vi "StartUp Sequence Open Loop Rev 1.2 -Retarded Engine Ramp Up.vi"() -> ()   [LabVIEW 2017]
panel:
  out "Turbine State 3":string
  out "Turbine State 2":string
  in  "Shut Off":bool
  out "ECU COM Port Out":refnum<visa-resource-name>
  out "Throttle Position":string
  out "Turbine RPM":string
  out "Turbine Temp":string
  out "Pump Voltage":string
  out "Error Out":errorcluster
  in  "Error In":errorcluster
  in  "ECU COM Port":refnum<visa-resource-name>
  out "Turbine State":string
  in  "Strt Sqnc":bool
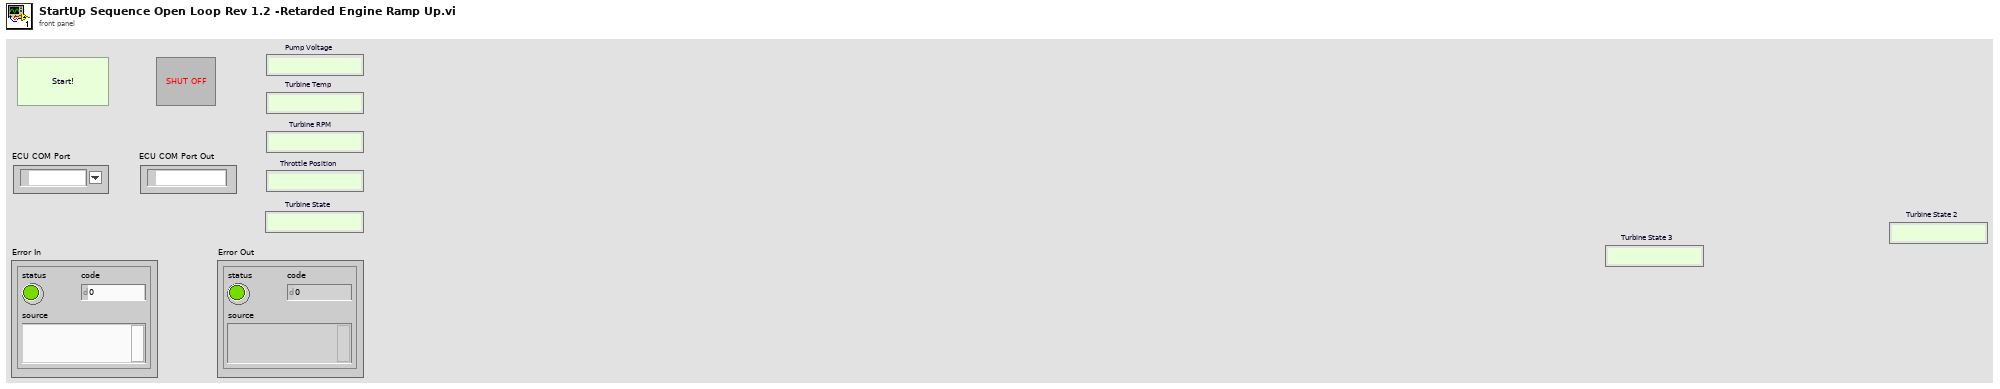
[diagram p1: front panel]
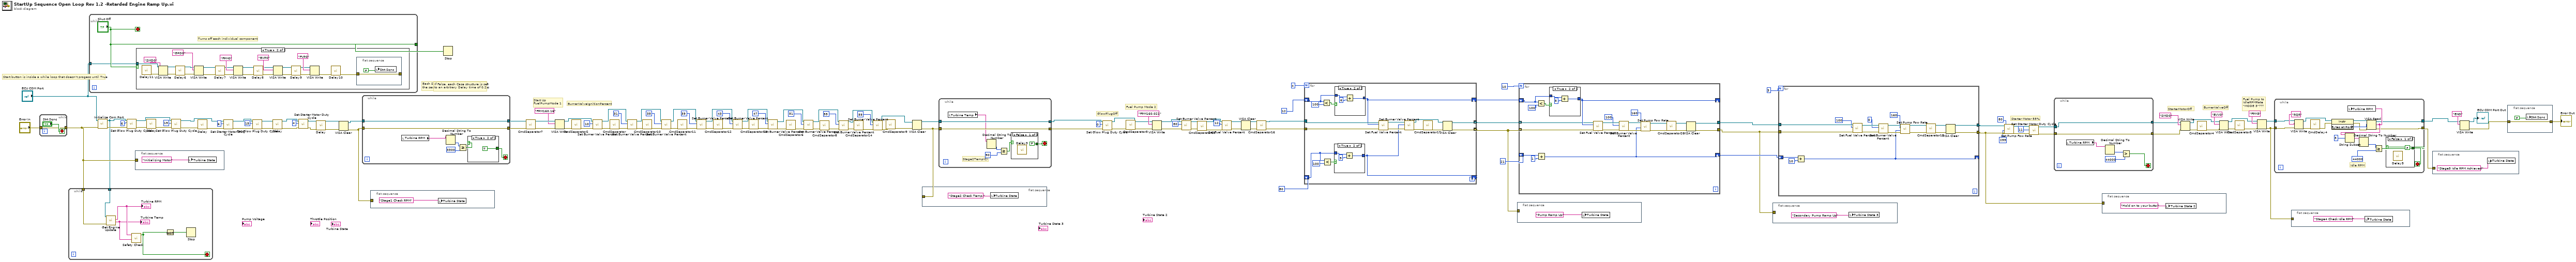
[diagram p0: block diagram]
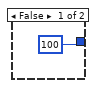
[diagram p2: hidden frame]
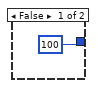
[diagram p3: hidden frame]
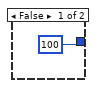
[diagram p4: hidden frame]
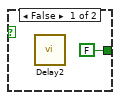
[diagram p6: hidden frame]
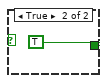
[diagram p7: hidden frame]
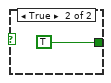
[diagram p8: hidden frame]
diagram:
  # "Starter Motor 55%"
  # "Start button is inside a while loop that doesn't progess until True"
  # "Fuel Pump Mode 2"
  # "Fuel Pump to \nIdleRPMRate\n\"MODE 3\"???"
  # "BurnerValveOff"
  # "StarterMotorOff"
  # "GlowPlugOff"
  # "Start Up\nFuelPumpMode 1"
  # "BurnerValveIgnitionPercent"
  # "If False, each Case structure is set\nto an arbitrary Delay time of 0.2 s"
  # "Each Stage is inside a while loop so that \nthe sequence doesn't progress until True"
  n1 = while {
    tunnel: "Error In" -> [w132]
    tunnel: [w132] -> w18
    stop <- "Strt Sqnc" stop-if-true
  }
  n2 = while {
    tunnel: ["Shut Off"] -> w104
    tunnel: "ECU COM Port" -> [w134]
    stop <- "Shut Off" stop-if-true
    # "Turns off each individual component"
    n3 = case shown="True" "Shut Off" {
      tunnel: w134 -> [_ w138]
      frame False {
      }
      frame True {
        n4 = call "Delay11"() -> ("error out"=w136:errorcluster)  [unwired: 11 in]
        n5 = VISA Write(VISA resource name=w138, write buffer="SMD0", error in (no error)=w136) -> (VISA resource name out=w143:refnum<visa-resource-name>, error out=w156:errorcluster)  [unwired: 1 out]
        n6 = call "Delay6"("error in (no error)"=w156) -> ("error out"=w150:errorcluster)  [unwired: 10 in]
        n7 = VISA Write(VISA resource name=w143, write buffer="GPD0", error in (no error)=w150) -> (VISA resource name out=w141:refnum<visa-resource-name>, error out=w154:errorcluster)  [unwired: 1 out]
        n8 = call "Delay7"("error in (no error)"=w154) -> ("error out"=w149:errorcluster)  [unwired: 10 in]
        n9 = VISA Write(VISA resource name=w141, write buffer="FPM0", error in (no error)=w149) -> (VISA resource name out=w140:refnum<visa-resource-name>, error out=w153:errorcluster)  [unwired: 1 out]
        n10 = call "Delay8"("error in (no error)"=w153) -> ("error out"=w148:errorcluster)  [unwired: 10 in]
        n11 = VISA Write(VISA resource name=w140, write buffer="BVP0", error in (no error)=w148) -> (VISA resource name out=w139:refnum<visa-resource-name>, error out=w152:errorcluster)  [unwired: 1 out]
        n12 = call "Delay9"("error in (no error)"=w152) -> ("error out"=w147:errorcluster)  [unwired: 10 in]
        n13 = VISA Write(VISA resource name=w139, write buffer="FVP0", error in (no error)=w147) -> (error out=w151:errorcluster)  [unwired: 2 out]
        n14 = call "Delay10"("error in (no error)"=w151) -> ("error out"=w137:errorcluster)  [unwired: 10 in]
        n15 = flat-sequence {
          tunnel: w137 -> [w157]
          tunnel: [w157] -> _
          frame #0 {
            n16 = local write "Strt Sqnc"(FALSE ("Strt Sqnc")) -> ()
          }
        }
      }
    }
  }
  n17 = call "Initialize Com Port.vi"("Error In"=w18, "ECU COM Port"="ECU COM Port") -> ("Error Out"=w92:errorcluster, "ECU COM Port Out"=w17:refnum<visa-resource-name>)  [unwired: 8 in]
  n18 = while {
    tunnel: w18 -> [w164]
    tunnel: w17 -> [w163]
    stop <- w160 stop-if-true
    n19 = call "Get Engine Update.vi"("Error In"=w164, "ECU COM Port"=w163) -> ("Temperature"=w161:string, "RPMs"=w162:string)  [unwired: 6 in, 2 out]
    "Turbine RPM" <- w162
    "Turbine Temp" <- w161
    n20 = call "Safety Check.vi"("Temperature"=w161, "RPMs"=w162) -> ("Safe?"=w160:bool)  [unwired: 9 in]
    n21 = Not(x=w160) -> (.not. x?=w159:bool)
    n22 = Stop(stop? (T)=w159) -> ()
  }
  n23 = call "Set Glow Plug Duty Cycle.vi"("Error In"=w92, "Duty Cycle"=6, "ECU COM Port"=w17) -> ("Error Out"=w91:errorcluster, "ECU COM Port Out"=w88:refnum<visa-resource-name>)  [unwired: 7 in]
  n24 = flat-sequence {
    tunnel: w18 -> [_]
    frame #0 {
      n25 = local write "Turbine State"("Initializing Motor") -> ()
    }
  }
  n26 = call "Delay"("error in (no error)"=w91) -> ("error out"=w90:errorcluster)  [unwired: 10 in]
  n27 = call "Set Glow Plug Duty Cycle.vi"("Error In"=w90, "Duty Cycle"=19, "ECU COM Port"=w88) -> ("Error Out"=w89:errorcluster, "ECU COM Port Out"=w84:refnum<visa-resource-name>)  [unwired: 7 in]
  n28 = call "Delay"("error in (no error)"=w89) -> ("error out"=w85:errorcluster)  [unwired: 10 in]
  n29 = call "Set Starter Motor Duty Cycle.vi"("Error In"=w85, "Duty Cycle"=6, "ECU COM Port"=w84) -> ("Error Out"=w83:errorcluster, "ECU COM Port Out"=w81:refnum<visa-resource-name>)  [unwired: 7 in]
  n30 = call "Set Glow Plug Duty Cycle.vi"("Error In"=w83, "Duty Cycle"=15, "ECU COM Port"=w81) -> ("Error Out"=w82:errorcluster, "ECU COM Port Out"=w77:refnum<visa-resource-name>)  [unwired: 7 in]
  n31 = call "Delay"("error in (no error)"=w82) -> ("error out"=w79:errorcluster)  [unwired: 10 in]
  n32 = call "Set Starter Motor Duty Cycle.vi"("Error In"=w79, "Duty Cycle"=4, "ECU COM Port"=w77) -> ("Error Out"=w78:errorcluster, "ECU COM Port Out"=w76:refnum<visa-resource-name>)  [unwired: 7 in]
  n33 = call "Delay"("error in (no error)"=w78) -> ("error out"=w107:errorcluster)  [unwired: 10 in]
  n34 = VISA Clear(VISA resource name=w76, error in (no error)=w107) -> (VISA resource name out=w108:refnum<visa-resource-name>, error out=w109:errorcluster)
  n35 = while {
    tunnel: w109 -> [w168]
    tunnel: w108 -> [w167]
    tunnel: [w167] -> w119
    tunnel: [w168] -> w118
    stop <- w171 stop-if-true
    n36 = local read "Turbine RPM"() -> (w166:string)
    n37 = Decimal String To Number(string=w166) -> (number=w170:i32)  [unwired: 2 in, 1 out]
    n38 = Greater Or Equal?(x=w170, y=3300) -> (x >= y?=w172:bool)
    n39 = case shown="True" w172 {
      tunnel: [FALSE TRUE] -> w171
      frame False {
        n40 = call "Delay2"() -> ()  [unwired: 11 in, 1 out]
      }
      frame True {
      }
    }
  }
  n41 = flat-sequence {
    tunnel: w109 -> [_]
    frame #0 {
      n42 = local write "Turbine State"("Stage1 Check RPM") -> ()
    }
  }
  n43 = Stop(stop? (T)=w104) -> ()
  n44 = call "CmdSeparator7"("error in (no error)"=w118) -> ("error out"=w117:errorcluster)  [unwired: 10 in]
  n45 = VISA Write(VISA resource name=w119, write buffer="FPM160,16", error in (no error)=w117) -> (VISA resource name out=w64:refnum<visa-resource-name>, error out=w130:errorcluster)  [unwired: 1 out]
  n46 = call "CmdSeparator2"("error in (no error)"=w130) -> ("error out"=w75:errorcluster)  [unwired: 10 in]
  n47 = call "Set Burner Valve Percent.vi"("Error In"=w75, "Percent"=10, "ECU COM Port"=w64) -> ("Error Out"=w74:errorcluster, "ECU COM Port Out"=w63:refnum<visa-resource-name>)  [unwired: 7 in]
  n48 = call "CmdSeparator"("error in (no error)"=w74) -> ("error out"=w73:errorcluster)  [unwired: 10 in]
  n49 = call "Set Burner Valve Percent.vi"("Error In"=w73, "Percent"=31, "ECU COM Port"=w63) -> ("Error Out"=w72:errorcluster, "ECU COM Port Out"=w62:refnum<visa-resource-name>)  [unwired: 7 in]
  n50 = call "CmdSeparator10"("error in (no error)"=w72) -> ("error out"=w71:errorcluster)  [unwired: 10 in]
  n51 = call "Set Burner Valve Percent.vi"("Error In"=w71, "Percent"=35, "ECU COM Port"=w62) -> ("Error Out"=w70:errorcluster, "ECU COM Port Out"=w61:refnum<visa-resource-name>)  [unwired: 7 in]
  n52 = call "CmdSeparator11"("error in (no error)"=w70) -> ("error out"=w69:errorcluster)  [unwired: 10 in]
  n53 = call "Set Burner Valve Percent.vi"("Error In"=w69, "Percent"=39, "ECU COM Port"=w61) -> ("Error Out"=w68:errorcluster, "ECU COM Port Out"=w60:refnum<visa-resource-name>)  [unwired: 7 in]
  n54 = call "CmdSeparator12"("error in (no error)"=w68) -> ("error out"=w67:errorcluster)  [unwired: 10 in]
  n55 = call "Set Burner Valve Percent.vi"("Error In"=w67, "Percent"=43, "ECU COM Port"=w60) -> ("Error Out"=w66:errorcluster, "ECU COM Port Out"=w59:refnum<visa-resource-name>)  [unwired: 7 in]
  n56 = call "CmdSeparator13"("error in (no error)"=w66) -> ("error out"=w65:errorcluster)  [unwired: 10 in]
  n57 = call "Set Burner Valve Percent.vi"("Error In"=w65, "Percent"=47, "ECU COM Port"=w59) -> ("Error Out"=w38:errorcluster, "ECU COM Port Out"=w37:refnum<visa-resource-name>)  [unwired: 7 in]
  n58 = call "CmdSeparator6"("error in (no error)"=w38) -> ("error out"=w40:errorcluster)  [unwired: 10 in]
  n59 = call "Set Burner Valve Percent.vi"("Error In"=w40, "Percent"=51, "ECU COM Port"=w37) -> ("Error Out"=w33:errorcluster, "ECU COM Port Out"=w34:refnum<visa-resource-name>)  [unwired: 7 in]
  n60 = call "CmdSeparator8"("error in (no error)"=w33) -> ("error out"=w36:errorcluster)  [unwired: 10 in]
  n61 = call "Set Burner Valve Percent.vi"("Error In"=w36, "Percent"=55, "ECU COM Port"=w34) -> ("Error Out"=w29:errorcluster, "ECU COM Port Out"=w30:refnum<visa-resource-name>)  [unwired: 7 in]
  n62 = call "CmdSeparator14"("error in (no error)"=w29) -> ("error out"=w32:errorcluster)  [unwired: 10 in]
  n63 = call "Set Burner Valve Percent.vi"("Error In"=w32, "Percent"=59, "ECU COM Port"=w30) -> ("Error Out"=w28:errorcluster, "ECU COM Port Out"=w27:refnum<visa-resource-name>)  [unwired: 7 in]
  n64 = call "CmdSeparator9"("error in (no error)"=w28) -> ("error out"=w103:errorcluster)  [unwired: 10 in]
  n65 = VISA Clear(VISA resource name=w27, error in (no error)=w103) -> (VISA resource name out=w105:refnum<visa-resource-name>, error out=w106:errorcluster)
  n66 = flat-sequence {
    tunnel: w106 -> [_]
    frame #0 {
      n67 = local write "Turbine State"("Stage2 Check Temp.") -> ()
    }
  }
  n68 = while {
    tunnel: w105 -> [w178]
    tunnel: w106 -> [w179]
    tunnel: [w178] -> w48
    tunnel: [w179] -> w49
    stop <- w182 stop-if-true
    # "Stage2Temp(C)"
    n69 = local read "Turbine Temp"() -> (w177:string)
    n70 = Decimal String To Number(string=w177) -> (number=w180:i32)  [unwired: 2 in, 1 out]
    n71 = Greater Or Equal?(x=w180, y=90) -> (x >= y?=w183:bool)
    n72 = case shown="False" w183 {
      tunnel: [FALSE TRUE] -> w182
      frame False {
        n73 = call "Delay3"() -> ()  [unwired: 11 in, 1 out]
      }
      frame True {
      }
    }
  }
  n74 = call "Set Glow Plug Duty Cycle.vi"("Error In"=w49, "Duty Cycle"=0, "ECU COM Port"=w48) -> ("Error Out"=w47:errorcluster, "ECU COM Port Out"=w45:refnum<visa-resource-name>)  [unwired: 7 in]
  n75 = call "CmdSeparator3"("error in (no error)"=w47) -> ("error out"=w46:errorcluster)  [unwired: 10 in]
  n76 = VISA Write(VISA resource name=w45, write buffer="FPM160,021", error in (no error)=w46) -> (VISA resource name out=w42:refnum<visa-resource-name>, error out=w44:errorcluster)  [unwired: 1 out]
  n77 = call "Set Burner Valve Percent.vi"("Error In"=w44, "Percent"=80, "ECU COM Port"=w42) -> ("Error Out"=w26:errorcluster, "ECU COM Port Out"=w41:refnum<visa-resource-name>)  [unwired: 7 in]
  n78 = call "CmdSeparator18"("error in (no error)"=w26) -> ("error out"=w25:errorcluster)  [unwired: 10 in]
  n79 = call "Set Fuel Valve Percent.vi"("Error In"=w25, "Percent"=12, "ECU COM Port"=w41) -> ("Error Out"=w24:errorcluster, "ECU COM Port Out"=w43:refnum<visa-resource-name>)  [unwired: 7 in]
  n80 = VISA Clear(VISA resource name=w43, error in (no error)=w24) -> (VISA resource name out=w99:refnum<visa-resource-name>, error out=w100:errorcluster)
  n81 = call "CmdSeparator16"("error in (no error)"=w100) -> ("error out"=w98:errorcluster)  [unwired: 10 in]
  n82 = for {
    N: 4 -> [_]
    tunnel: [w186] -> _
    tunnel: [w187] -> _
    tunnel: w99 -> [w194]
    tunnel: w98 -> [w195]
    shift-right: [w193] -> w20
    shift-left: 12 -> [w199]
    shift-right: [w190] -> _
    shift-left: 80 -> [w196]
    tunnel: [w187] -> w7 mode=indexing
    tunnel: [w186] -> w21 mode=indexing
    n83 = Less?(x=w199, y=100) -> (x < y?=w200:bool)
    n84 = Less?(x=w196, y=100) -> (x < y?=w197:bool)
    n85 = case shown="True" w197 {
      tunnel: w196 -> [_ w206]
      tunnel: [100 w204] -> w190
      frame False {
      }
      frame True {
        n86 = Add(x=w206, y=5) -> (x+y=w204:i32)
      }
    }
    n87 = case shown="True" w200 {
      tunnel: w199 -> [_ w210]
      tunnel: [100 w208] -> w193
      frame False {
      }
      frame True {
        n88 = Add(x=w210, y=6) -> (x+y=w208:i32)
      }
    }
    n89 = call "Set Fuel Valve Percent.vi"("Error In"=w195, "Percent"=w193, "ECU COM Port"=w194) -> ("Error Out"=w192:errorcluster, "ECU COM Port Out"=w189:refnum<visa-resource-name>)  [unwired: 7 in]
    n90 = call "Set Burner Valve Percent.vi"("Error In"=w192, "Percent"=w190, "ECU COM Port"=w189) -> ("Error Out"=w191:errorcluster, "ECU COM Port Out"=w188:refnum<visa-resource-name>)  [unwired: 7 in]
    n91 = call "CmdSeparator17"("error in (no error)"=w191) -> ("error out"=w202:errorcluster)  [unwired: 10 in]
    n92 = VISA Clear(VISA resource name=w188, error in (no error)=w202) -> (VISA resource name out=w186:refnum<visa-resource-name>, error out=w187:errorcluster)
  }
  n93 = flat-sequence {
    tunnel: w7 -> [_]
    frame #0 {
      n94 = local write "Turbine State"("Pump Ramp Up") -> ()
    }
  }
  n95 = for {
    N: 10 -> [_]
    tunnel: [w223] -> w15
    tunnel: [w224] -> w6
    shift-right: [w227] -> _
    shift-left: w20 -> [w228]
    tunnel: w7 -> [w222] mode=indexing
    tunnel: w21 -> [w221] mode=indexing
    shift-right: [w212] -> w14
    shift-left: 21 -> [w213]
    n96 = Less?(x=w228, y=100) -> (x < y?=w229:bool)
    n97 = Add(x=w213, y=1) -> (x+y=w212:i32)
    n98 = case shown="True" w229 {
      tunnel: w228 -> [_ w235]
      tunnel: [100 w233] -> w227
      frame False {
      }
      frame True {
        n99 = Add(x=w235, y=5) -> (x+y=w233:i32)
      }
    }
    n100 = call "Set Fuel Valve Percent.vi"("Error In"=w222, "Percent"=w227, "ECU COM Port"=w221) -> ("Error Out"=w226:errorcluster, "ECU COM Port Out"=w225:refnum<visa-resource-name>)  [unwired: 7 in]
    n101 = call "Set Burner Valve Percent.vi"("Error In"=w226, "Percent"=100 ("y"), "ECU COM Port"=w225) -> ("Error Out"=w216:errorcluster, "ECU COM Port Out"=w219:refnum<visa-resource-name>)  [unwired: 7 in]
    n102 = call "Set Pump Fow Rate.vi"("Error In"=w216, "Pulse Width"=w212, "Voltage"=160 ("y"), "ECU COM Port"=w219) -> ("Error Out"=w217:errorcluster, "ECU COM Port Out"=w218:refnum<visa-resource-name>)  [unwired: 6 in]
    n103 = call "CmdSeparator20"("error in (no error)"=w217) -> ("error out"=w231:errorcluster)  [unwired: 10 in]
    n104 = VISA Clear(VISA resource name=w218, error in (no error)=w231) -> (VISA resource name out=w223:refnum<visa-resource-name>, error out=w224:errorcluster)
  }
  n105 = flat-sequence {
    tunnel: w6 -> [_]
    frame #0 {
      n106 = local write "Turbine State 3"("Secondary Pump Ramp Up") -> ()
    }
  }
  n107 = for {
    N: 3 -> [_]
    tunnel: [w249] -> w10
    tunnel: [w250] -> w5
    tunnel: w6 -> [w248]
    tunnel: w15 -> [w247]
    shift-right: [w238] -> _
    shift-left: w14 -> [w239]
    n108 = Add(x=w239, y=10) -> (x+y=w238:i32)
    n109 = call "Set Fuel Valve Percent.vi"("Error In"=w248, "Percent"=100 ("y"), "ECU COM Port"=w247) -> ("Error Out"=w252:errorcluster, "ECU COM Port Out"=w251:refnum<visa-resource-name>)  [unwired: 7 in]
    n110 = call "Set Burner Valve Percent.vi"("Error In"=w252, "Percent"=0 ("y"), "ECU COM Port"=w251) -> ("Error Out"=w242:errorcluster, "ECU COM Port Out"=w245:refnum<visa-resource-name>)  [unwired: 7 in]
    n111 = call "Set Pump Fow Rate.vi"("Error In"=w242, "Pulse Width"=w238, "Voltage"=160 ("y"), "ECU COM Port"=w245) -> ("Error Out"=w243:errorcluster, "ECU COM Port Out"=w244:refnum<visa-resource-name>)  [unwired: 6 in]
    n112 = call "CmdSeparator15"("error in (no error)"=w243) -> ("error out"=w253:errorcluster)  [unwired: 10 in]
    n113 = VISA Clear(VISA resource name=w244, error in (no error)=w253) -> (VISA resource name out=w249:refnum<visa-resource-name>, error out=w250:errorcluster)
  }
  n114 = call "Set Pump Fow Rate.vi"("Error In"=w5, "Pulse Width"=255, "Voltage"=80, "ECU COM Port"=w10) -> ("Error Out"=w11:errorcluster, "ECU COM Port Out"=w12:refnum<visa-resource-name>)  [unwired: 6 in]
  n115 = call "Set Starter Motor Duty Cycle.vi"("Error In"=w11, "Duty Cycle"=11, "ECU COM Port"=w12) -> ("Error Out"=w4:errorcluster, "ECU COM Port Out"=w3:refnum<visa-resource-name>)  [unwired: 7 in]
  n116 = while {
    tunnel: w4 -> [w255]
    tunnel: w3 -> [w254]
    tunnel: [w255] -> w2
    tunnel: [w254] -> w1
    stop <- w256 stop-if-true
    n117 = local read "Turbine RPM"() -> (w259:string)
    n118 = Decimal String To Number(string=w259) -> (number=w258:i32)  [unwired: 2 in, 1 out]
    n119 = Greater?(x=w258, y=44000) -> (0:w256:bool)
  }
  n120 = flat-sequence {
    tunnel: w5 -> [_]
    frame #0 {
      n121 = local write "Turbine State 2"("Hold on to your butts!") -> ()
    }
  }
  n122 = VISA Write(VISA resource name=w1, write buffer="SMD0", error in (no error)=w2) -> (VISA resource name out=w125:refnum<visa-resource-name>, error out=w127:errorcluster)  [unwired: 1 out]
  n123 = call "CmdSeparator4"("error in (no error)"=w127) -> ("error out"=w126:errorcluster)  [unwired: 10 in]
  n124 = VISA Write(VISA resource name=w125, write buffer="BVV0", error in (no error)=w126) -> (VISA resource name out=w122:refnum<visa-resource-name>, error out=w121:errorcluster)  [unwired: 1 out]
  n125 = call "CmdSeparator5"("error in (no error)"=w121) -> ("error out"=w123:errorcluster)  [unwired: 10 in]
  n126 = VISA Write(VISA resource name=w122, write buffer="FPM3", error in (no error)=w123) -> (VISA resource name out=w120:refnum<visa-resource-name>, error out=w111:errorcluster)  [unwired: 1 out]
  n127 = while {
    tunnel: w120 -> [w267]
    tunnel: w111 -> [w266]
    tunnel: [w264] -> w110
    tunnel: [w263] -> w113
    stop <- w278 stop-if-true
    # "Idle RPM"
    n128 = VISA Write(VISA resource name=w267, write buffer="RQR", error in (no error)=w266) -> (VISA resource name out=w274:refnum<visa-resource-name>, error out=w276:errorcluster)  [unwired: 1 out]
    n129 = call "CmdDelay4"("error in (no error)"=w276) -> ("error out"=w275:errorcluster)  [unwired: 10 in]
    n130 = property class="Instr"(reference=w274, error in=w275) -> (reference out=w271:refnum<visa-resource-name>, error out=w272:errorcluster, "Bytes at Port"=w273:u32)
    n131 = VISA Read(VISA resource name=w271, byte count=w273, error in (no error)=w272) -> (VISA resource name out=w263:refnum<visa-resource-name>, read buffer=w265:string, error out=w264:errorcluster)  [unwired: 1 out]
    n132 = String Subset(string=w265, offset (0)=3) -> (substring=w269:string)  [unwired: 1 in]
    n133 = local write "Turbine RPM"(w265) -> ()
    n134 = Decimal String To Number(string=w269) -> (number=w268:i32)  [unwired: 2 in, 1 out]
    n135 = Greater Or Equal?(x=w268, y=44000) -> (x >= y?=w262:bool)
    n136 = case shown="False" w262 {
      tunnel: [FALSE TRUE] -> w278
      frame False {
        n137 = call "Delay5"() -> ()  [unwired: 11 in, 1 out]
      }
      frame True {
      }
    }
  }
  n138 = flat-sequence {
    tunnel: w111 -> [_]
    frame #0 {
      n139 = local write "Turbine State"("Stage4 Check Idle RPM") -> ()
    }
  }
  n140 = flat-sequence {
    tunnel: w110 -> [_]
    frame #0 {
      n141 = local write "Turbine State"("Stage5 Idle RPM Achieved") -> ()
    }
  }
  n142 = VISA Write(VISA resource name=w113, write buffer="END") -> (VISA resource name out=→"ECU COM Port Out":refnum<visa-resource-name>, error out=w102:errorcluster)  [unwired: 1 in, 1 out]
  n143 = flat-sequence {
    tunnel: w102 -> [w283]
    tunnel: [w283] -> w101
    frame #0 {
      n144 = local write "Strt Sqnc"(FALSE ("Strt Sqnc")) -> ()
    }
  }
  "Error Out" <- w101
